vi "MultiColumnListbox_Resize.vi"(7 "Parent VI Reference":refnum<vi>, 8 "error in (no error)":errorcluster, 9 "Fit to pane?":bool, 10 "Column Widths [%]":u32[](array[numeric]), 11 "MCListbox Refnum":refnum<vi>) -> (0 "error out":errorcluster)   [LabVIEW 2022 SP3, in "hse-ui.lvlib"]
doc: "Resizes the columns of a MCLB according to the widths given in <b>Column Widths [%]</b>. If <b>Parent VI Reference</b> is supplied, panel updates are deferred.\n\n____\nHAMPEL SOFTWARE ENGINEERING v3.8.0 (2023-12-18 14:41)"
uses:
  hse-ui.lvlib
  <vilib>/Utility/miscctls.llb/LVRowAndColumnTypeDef.ctl
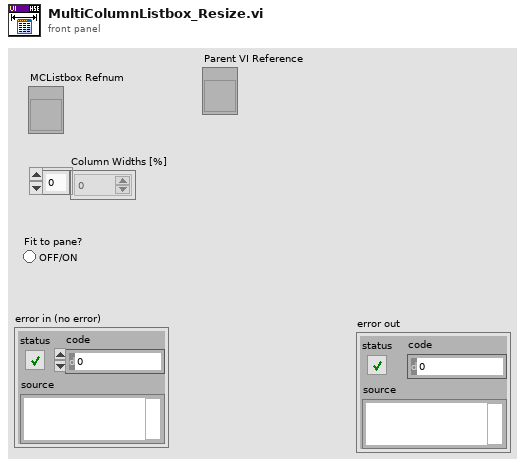
[diagram p1: front panel]
types:
  T1 = typedef "LVRowAndColumnTypeDef.ctl" = cluster{"Row":i32, "Column":i32}
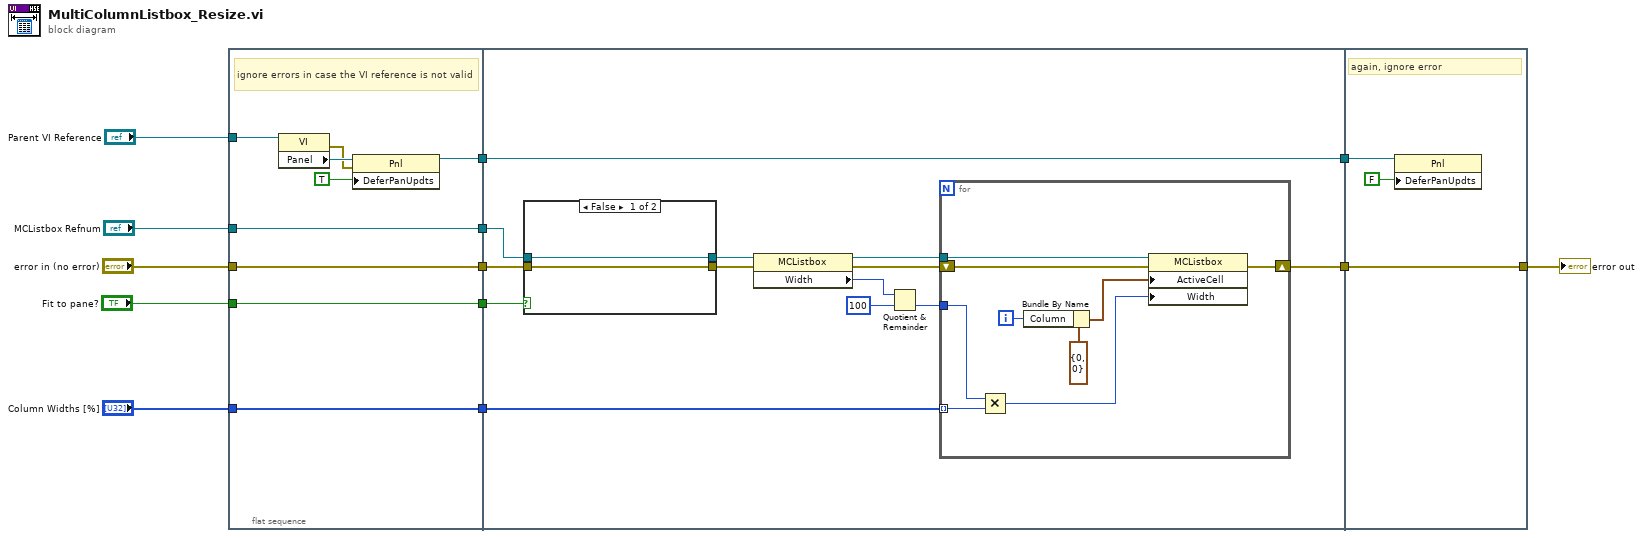
[diagram p0: block diagram]
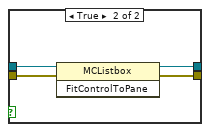
[diagram p2: hidden frame]
diagram:
  n1 = flat-sequence {
    tunnel: "Fit to pane?" -> [w19]
    tunnel: "error in (no error)" -> [w20]
    tunnel: "Column Widths [%]" -> [w21]
    tunnel: "MCListbox Refnum" -> [w22]
    tunnel: [w22] -> w8
    tunnel: [w21] -> w7
    tunnel: [w20] -> w6
    tunnel: [w19] -> w5
    tunnel: "Parent VI Reference" -> [w15]
    tunnel: [w14] -> w3
    tunnel: [w25] -> w9
    tunnel: w8 -> [w35]
    tunnel: w7 -> [w28]
    tunnel: w6 -> [w27]
    tunnel: w5 -> [w24]
    tunnel: [w23] -> w4
    tunnel: w3 -> [w23]
    tunnel: [w53] -> w11
    tunnel: w9 -> [w53]
    tunnel: w4 -> [w51]
    frame #0 {
      # "ignore errors in case the VI reference is not valid"
      n2 = property class="VI"(reference=w15) -> (error out=w17:errorcluster, "Panel"=w18:refnum<vi>)  [unwired: 1 in, 1 out]
      n3 = property class="Pnl"(reference=w18, error in=w17, "DeferPanUpdts"=TRUE ("Defer Panel Updates")) -> (reference out=w14:refnum<vi>)  [unwired: 1 out]
    }
    frame #1 {
      n4 = case shown="False" w24 {
        tunnel: w35 -> [w37 w41]
        tunnel: [w36 w40] -> w32
        tunnel: [w37 w39] -> w31
        tunnel: w27 -> [w36 w38]
        frame False {
        }
        frame True {
          n5 = invoke class="MCListbox" method="FitControlToPane"(reference=w41, error in=w38) -> (reference out=w39:refnum<vi>, error out=w40:errorcluster)  [unwired: 1 in, 1 out]
        }
      }
      n6 = property on="Property Node" class="MCListbox"(reference=w31, error in=w32) -> (reference out=w34:refnum<vi>, error out=w26:errorcluster, "Width"=w33:u32)
      n7 = Quotient & Remainder(x=w33, y=u32 100) -> (floor(x/y)=w29:u32)  [unwired: 1 out]
      n8 = for {
        tunnel: w29 -> [w48]
        tunnel: w28 -> [w47] mode=indexing
        tunnel: w34 -> [w44]
        shift-right: [w42] -> w25
        shift-left: w26 -> [w43]
        i -> [w45]
        n9 = Multiply(x=w48, y=w47) -> (x*y=w46:u32)
        n10 = Bundle By Name(cluster=T1 {"Row"=0, "Column"=0} ("Active Cell:Active Cell"), "Column"=w45) -> (w49:T1)
        n11 = property on="Property Node" class="MCListbox"(reference=w44, error in=w43, "ActiveCell"=w49, "Width"=w46) -> (error out=w42:errorcluster)  [unwired: 1 out]
      }
    }
    frame #2 {
      # "again, ignore error"
      n12 = property class="Pnl"(reference=w51, "DeferPanUpdts"=FALSE ("Defer Panel Updates")) -> ()  [unwired: 1 in, 2 out]
    }
  }
  "error out" <- w11
